vi "Swerve Math (SubVI).vi"(1 "Wheelbase (L)":dbl, 2 "Trackwidth (W)":dbl, 11 "Joystick Input":T3 {"Joystick 2 X (Rotate)" scale=1.0..-1.0; "Joystick 1 Y (forward/back)" scale=-1.0..1.0; "Joystick 1 X (strafe)" scale=1.0..-1.0}, 12 "Gyro Angle in degrees":dbl) -> (4 "wheelPowerDesired":T2, 15 "wheelAngleDesired(-180..180)":T1)   [LabVIEW 2020]
uses:
  TypeDefs/Joysticks.ctl
  TypeDefs/WheelAngleDesired.ctl
  TypeDefs/WheelPowerDesired.ctl
panel:
  in  "wheelPowerDesired":T2
  in  "wheelAngleDesired(-180..180)":T1
  out "LFW":dbl(knob) scale=180.0..-180.0
  out "RFW":dbl(knob) scale=180.0..-180.0
  out "RRW":dbl(knob) scale=180.0..-180.0
  out "LRW":dbl(knob) scale=180.0..-180.0
  # "Inputs"
  # "Front of Robot"
  # "Rear of Robot"
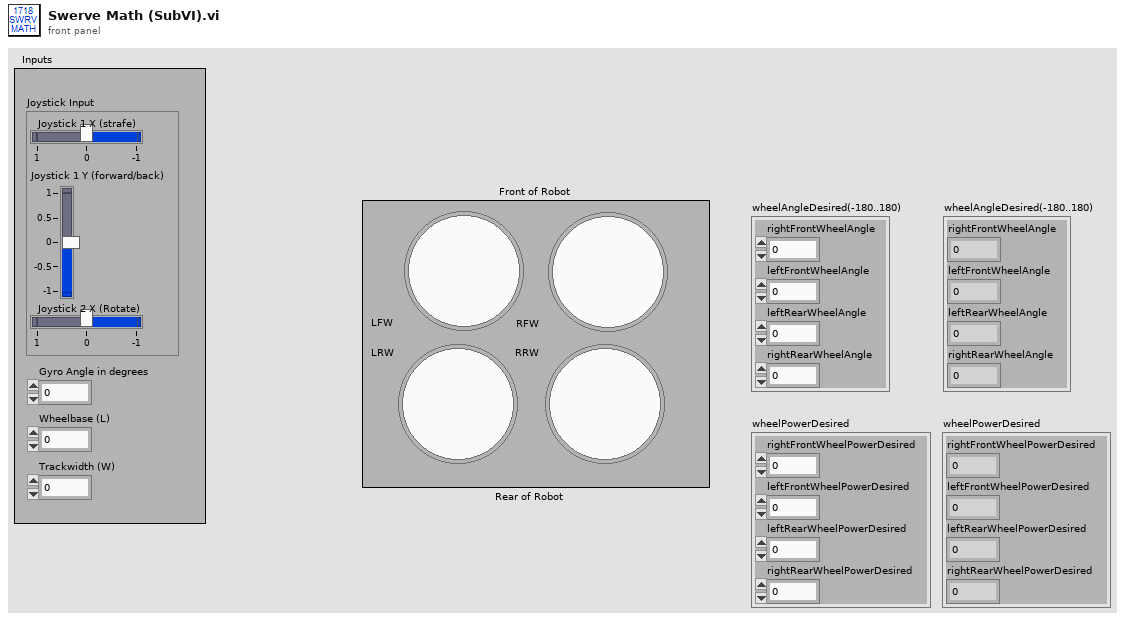
[diagram p1: front panel]
types:
  T1 = typedef "WheelAngleDesired.ctl" = cluster{"rightFrontWheelAngle":dbl, "leftFrontWheelAngle":dbl, "leftRearWheelAngle":dbl, "rightRearWheelAngle":dbl}
  T2 = typedef "WheelPowerDesired.ctl" = cluster{"rightFrontWheelPowerDesired":dbl, "leftFrontWheelPowerDesired":dbl, "leftRearWheelPowerDesired":dbl, "rightRearWheelPowerDesired":dbl}
  T3 = typedef "Joysticks.ctl" = cluster{"Joystick 1 X (strafe)":dbl, "Joystick 1 Y (forward/back)":dbl, "Joystick 2 X (Rotate)":dbl}
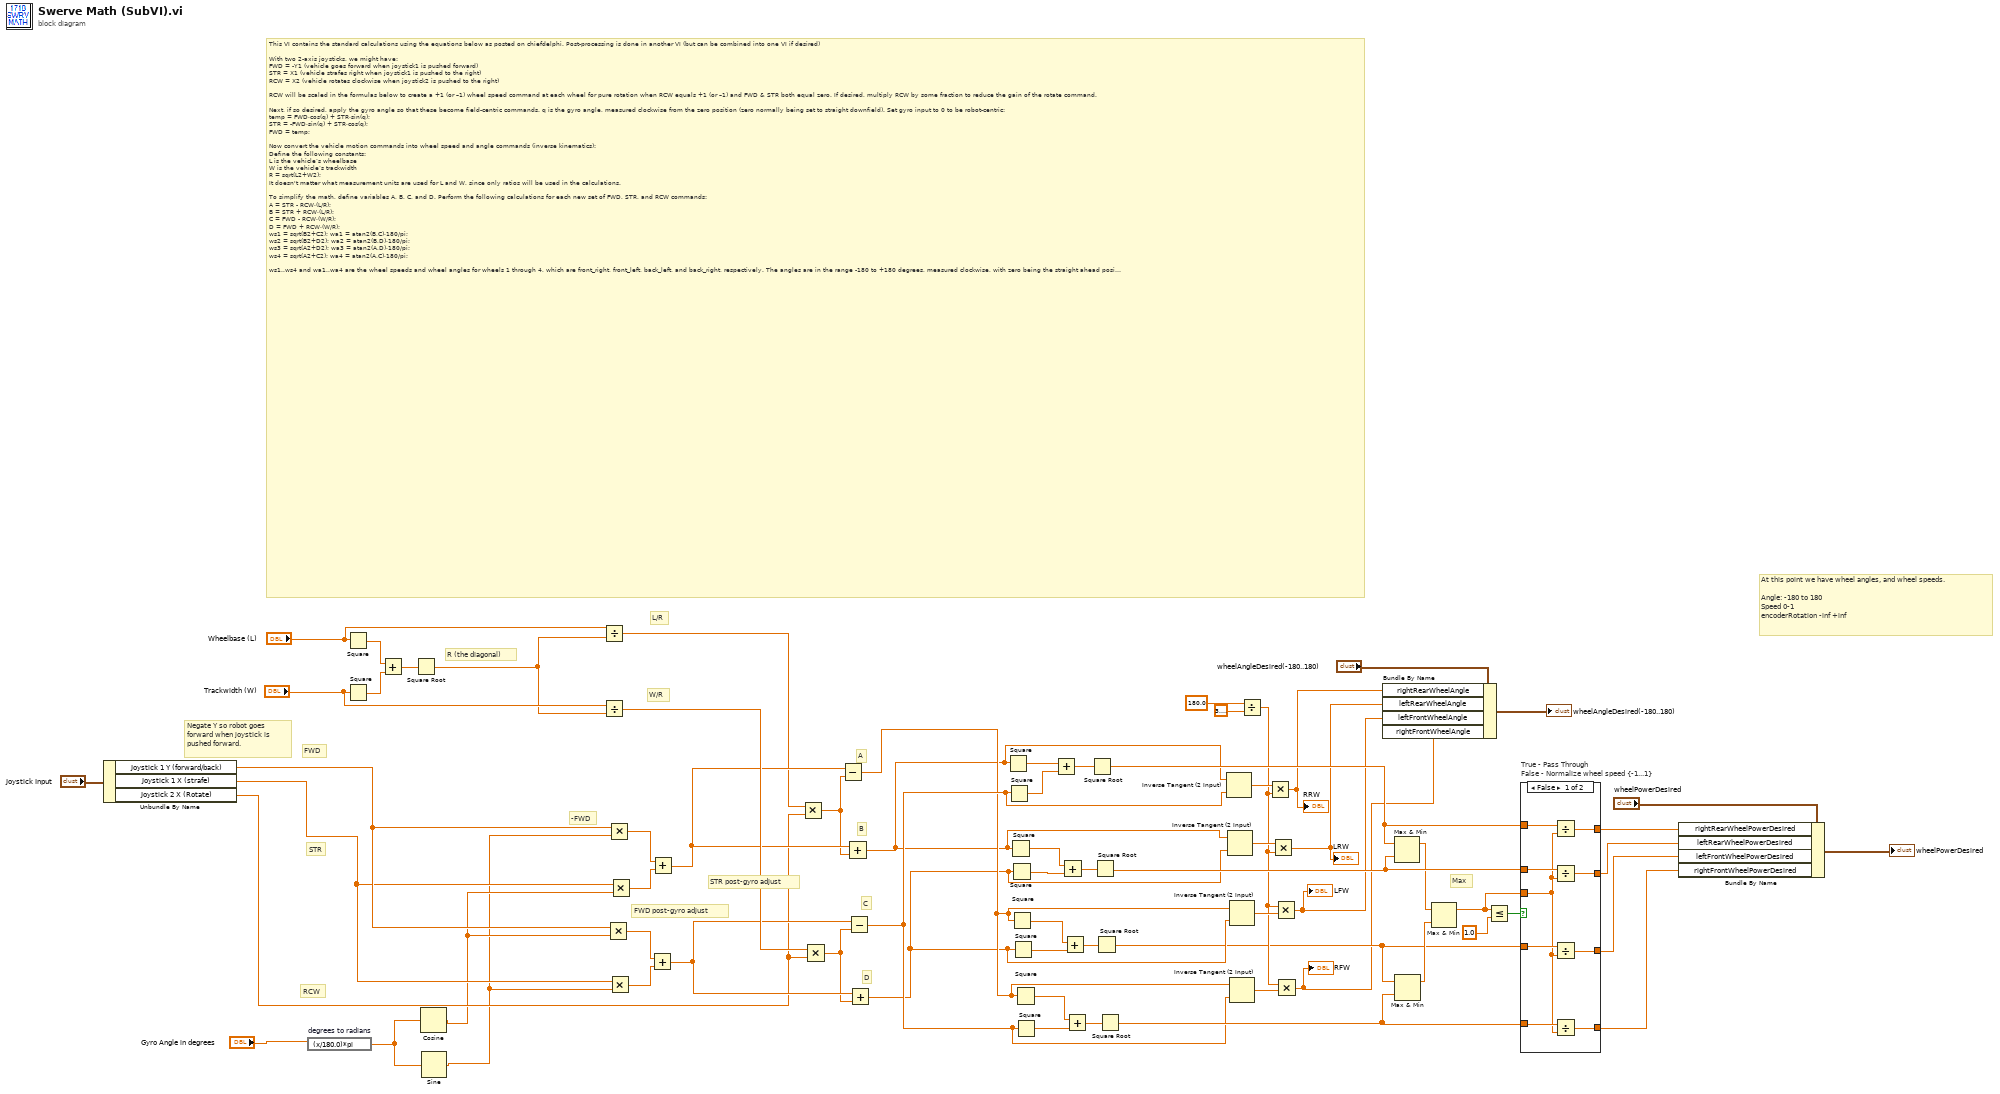
[diagram p0: block diagram]
diagram:
  # "At this point we have wheel angles, and wheel speeds.\n\nAngle: -180 to 180\nSpeed 0-1\nencoderRotation -inf +inf"
  # "This VI contains the standard calculations using the equations below as posted on chiefdelphi. Post-processing is done in another VI (but can be combined into one VI if desired)\n\nWith two 2-axis joysticks, we might have:\nFWD = -Y1 (vehicle goes forward when joystick1 is pushed forward)\nSTR = X1 (vehicle strafes right when joystick1 is pushed to the right)\nRCW = X2 (vehicle rotates clockwise when joystick2 is pushed to the right)\n\nRCW will be scaled in the formulas below to create a +1 (or –1) wheel speed command at each wheel for pure rotation when RCW equals +1 (or –1) and FWD & STR both equal zero. If desired, multiply RCW by some fraction to reduce the gain of the rotate command.\n\nNext, if so desired, apply the gyro angle so that these become field-centric commands. q is the gyro angle, measured clockwise from the zero position (zero normally being set to straight downfield). Set gyro input to 0 to be robot-centric:\ntemp = FWD·cos(q) + STR·sin(q);\nSTR = -FWD·sin(q) + STR·cos(q);\nFWD = temp;\n\nNow convert the vehicle motion commands into wheel speed and angle commands (inverse kinematics):\nDefine the following constants:\nL is the vehicle’s wheelbase\nW is the vehicle’s trackwidth\nR = sqrt(L2+W2);\nIt doesn't matter what measurement units are used for L and W, since only ratios will be used in the calculations.\n\nTo simplify the math, define variables A, B, C, and D. Perform the following calculations for each new set of FWD, STR, and RCW commands:\nA = STR - RCW·(L/R);\nB = STR + RCW·(L/R);\nC = FWD - RCW·(W/R);\nD = FWD + RCW·(W/R);\nws1 = sqrt(B2+C2); wa1 = atan2(B,C)·180/pi;\nws2 = sqrt(B2+D2); wa2 = atan2(B,D)·180/pi;\nws3 = sqrt(A2+D2); wa3 = atan2(A,D)·180/pi;\nws4 = sqrt(A2+C2); wa4 = atan2(A,C)·180/pi;\n\nws1..ws4 and wa1..wa4 are the wheel speeds and wheel angles for wheels 1 through 4, which are front_right, front_left, back_left, and back_right, respectively. The angles are in the range -180 to +180 degrees, measured clockwise, with zero being the straight ahead position. The wheel speeds need to be normalized before being used, as follows:\nmax = the largest of ws1, ws2, ws3, ws4 \nif (max >1) {ws1/=max; ws2/=max; ws3/=max; ws4/=max;} \n\nThe 4 wheel speeds are now in the range 0 to +1. Notice 0 to +1 and not -1 to +1, because each speed is always in the direction of the corresponding wheel angle. The 4 wheel speed and wheel angle pairs are now suitable for sending to a control algorithm which will decide how to actuate the steering and drive motors to achieve those speeds and angles for each wheel.\n\nThis is a separate and interesting problem, which may involve, for example, logic to reverse the wheel speed instead of steering the wheel 180 degrees (and similarly for other steering/speed commands). This control logic is highly dependent on the limitations of the vehicle design, such as the response of the steering motor, and the fact that some vehicles may have limitless steering (coaxial or slip rings) whereas others may be steering-limited. More complex logic may also take into account the current vehicle speed and recent past history in innovative ways. Computing the necessary speed and angle errors to send to a PID control (for example) may therefore become a non-trivial task in an effort to achieve smooth and seamless control."
  # "-FWD"
  # "Negate Y so robot goes\nforward when joystick is\npushed forward."
  # "Max"
  # "A"
  # "B"
  # "C"
  # "D"
  # "STR post-gyro adjust"
  # "FWD post-gyro adjust"
  # "RCW"
  # "STR"
  # "FWD"
  # "R (the diagonal)"
  # "W/R"
  # "L/R"
  n1 = Unbundle By Name("Joystick Input") -> ("Joystick 1 Y (forward/back)"=w11:dbl, "Joystick 1 X (strafe)"=w10:dbl, "Joystick 2 X (Rotate)"=w19:dbl)
  n2 = expression code="(x/180.0)*pi" "degrees to radians"("Gyro Angle in degrees") -> (w24:dbl)
  n3 = Square(x="Wheelbase (L)") -> (x^2=w26:dbl)
  n4 = Square(x="Trackwidth (W)") -> (x^2=w27:dbl)
  n5 = Add(x=w26, y=w27) -> (x+y=w28:dbl)
  n6 = Square Root(x=w28) -> (sqrt(x)=w25:dbl)
  n7 = Cosine(x=w24) -> (cos(x)=w2:dbl)
  n8 = Sine(x=w24) -> (sin(x)=w1:dbl)
  n9 = Divide(x="Wheelbase (L)", y=w25) -> (x/y=w35:dbl)
  n10 = Divide(x="Trackwidth (W)", y=w25) -> (x/y=w38:dbl)
  n11 = Multiply(x=w11, y=w2) -> (x*y=w29:dbl)
  n12 = Multiply(x=w11, y=w1) -> (x*y=w31:dbl)
  n13 = Multiply(x=w10, y=w1) -> (x*y=w30:dbl)
  n14 = Multiply(x=w10, y=w2) -> (x*y=w32:dbl)
  n15 = Add(x=w29, y=w30) -> (x+y=w37:dbl)
  n16 = Add(x=w31, y=w32) -> (x+y=w36:dbl)
  n17 = Multiply(x=w35, y=w19) -> (x*y=w23:dbl)
  n18 = Multiply(x=w38, y=w19) -> (x*y=w22:dbl)
  n19 = Subtract(x=w36, y=w23) -> (x-y=w59:dbl)
  n20 = Add(x=w36, y=w23) -> (x+y=w17:dbl)
  n21 = Subtract(x=w37, y=w22) -> (x-y=w60:dbl)
  n22 = Add(x=w37, y=w22) -> (x+y=w58:dbl)
  n23 = Square(x=w17) -> (x^2=w43:dbl)
  n24 = Square(x=w60) -> (x^2=w44:dbl)
  n25 = Square(x=w17) -> (x^2=w45:dbl)
  n26 = Square(x=w58) -> (x^2=w46:dbl)
  n27 = Square(x=w59) -> (x^2=w47:dbl)
  n28 = Square(x=w58) -> (x^2=w48:dbl)
  n29 = Square(x=w59) -> (x^2=w49:dbl)
  n30 = Square(x=w60) -> (x^2=w50:dbl)
  n31 = Add(x=w43, y=w44) -> (x+y=w39:dbl)
  n32 = Add(x=w45, y=w46) -> (x+y=w40:dbl)
  n33 = Add(x=w47, y=w48) -> (x+y=w41:dbl)
  n34 = Add(x=w49, y=w50) -> (x+y=w42:dbl)
  n35 = Square Root(x=w39) -> (sqrt(x)=w65:dbl)
  n36 = Square Root(x=w40) -> (sqrt(x)=w66:dbl)
  n37 = Square Root(x=w41) -> (sqrt(x)=w21:dbl)
  n38 = Square Root(x=w42) -> (sqrt(x)=w67:dbl)
  n39 = Inverse Tangent (2 Input)(1:w60, 2:w17) -> (0:w57:dbl)
  n40 = Inverse Tangent (2 Input)(1:w58, 2:w17) -> (0:w56:dbl)
  n41 = Inverse Tangent (2 Input)(1:w58, 2:w59) -> (0:w55:dbl)
  n42 = Inverse Tangent (2 Input)(1:w60, 2:w59) -> (0:w54:dbl)
  n43 = Divide(x=180.0, y=3.141592653589793) -> (x/y=w53:dbl)
  n44 = Multiply(x=w57, y=w53) -> (x*y=w6:dbl)
  "RRW" <- w6
  n45 = Multiply(x=w56, y=w53) -> (x*y=w5:dbl)
  "LRW" <- w5
  n46 = Multiply(x=w53, y=w55) -> (x*y=w4:dbl)
  "LFW" <- w4
  n47 = Multiply(x=w53, y=w54) -> (x*y=w3:dbl)
  "RFW" <- w3
  n48 = Bundle By Name(cluster="wheelAngleDesired(-180..180)", "rightRearWheelAngle"=w6, "leftRearWheelAngle"=w5, "leftFrontWheelAngle"=w4, "rightFrontWheelAngle"=w3) -> (→"wheelAngleDesired(-180..180)":T1)
  n49 = Max & Min(x=w65, y=w66) -> (max(x,y)=w62:dbl)  [unwired: 1 out]
  n50 = Max & Min(x=w21, y=w67) -> (max(x,y)=w61:dbl)  [unwired: 1 out]
  n51 = Max & Min(x=w62, y=w61) -> (max(x,y)=w68:dbl)  [unwired: 1 out]
  n52 = Less Or Equal?(x=w68, y=1.0) -> (x <= y?=w63:bool)
  n53 = case "True - Pass Through\nFalse - Normalize wheel speed {-1...1}" shown="False" w63 {
    tunnel: w65 -> [w74 w81]
    tunnel: w66 -> [w75 w80]
    tunnel: w21 -> [w77 w79]
    tunnel: w67 -> [w76 w78]
    tunnel: w68 -> [w73 _]
    tunnel: [w72 w81] -> w15
    tunnel: [w71 w80] -> w14
    tunnel: [w70 w79] -> w13
    tunnel: [w69 w78] -> w12
    frame False {
      n54 = Divide(x=w74, y=w73) -> (x/y=w72:dbl)
      n55 = Divide(x=w75, y=w73) -> (x/y=w71:dbl)
      n56 = Divide(x=w77, y=w73) -> (x/y=w70:dbl)
      n57 = Divide(x=w76, y=w73) -> (x/y=w69:dbl)
    }
    frame True {
    }
  }
  n58 = Bundle By Name(cluster="wheelPowerDesired", "rightRearWheelPowerDesired"=w15, "leftRearWheelPowerDesired"=w14, "leftFrontWheelPowerDesired"=w13, "rightFrontWheelPowerDesired"=w12) -> (→"wheelPowerDesired":T2)
